vi "ifr2025 Sweep Mode.vi"(5 "Sweep Type (Linear)":bool=TRUE, 6 "Trigger Source (Front Panel)":i16(ring)=10 items=["Hold", "TTLTRG0", "TTLTRG1", "TTLTRG2", "TTLTRG3", "TTLTRG4", "TTLTRG5", "TTLTRG6", "TTLTRG7", "BUS", "Front Panel"], 7 "Trigger mode (Start Only)":i16(ring)=1 items=["Off", "Start Only", "Start / Stop", "Step"], 8 "error in (no error)":errorcluster {"code" format="%.0x"}, 9 "Sweep Mode (Single)":bool=TRUE, 10 "Carr Freq (Fixed)":bool=TRUE, 11 "instrument handle":refnum<visa-resource-name>) -> (0 "error out":errorcluster {"code" format="%.0x"}, 3 "instrument handle out":refnum<visa-resource-name>)   [LabVIEW 2009]
doc: "This command defines the carrier mode (SWEPT or FIXED) and the remainder of the SWEPT mode parameters."
uses:
  Ifr2025_32.dll
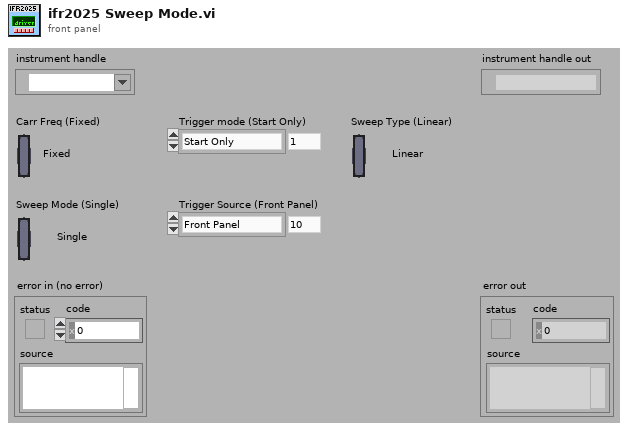
[diagram p1: front panel]
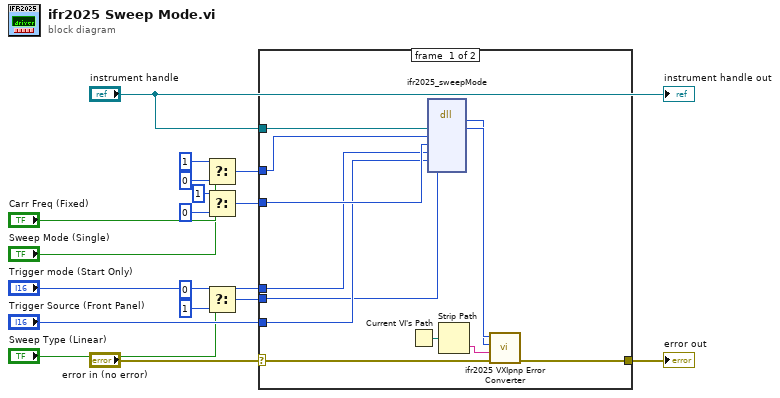
[diagram p0: block diagram]
diagram:
  n1 = Select(t=i16 1, s="Carr Freq (Fixed)", f=i16 0) -> (s? t:f=w11:i16)
  n2 = Select(t=i16 1, s="Sweep Mode (Single)", f=i16 0) -> (s? t:f=w7:i16)
  n3 = Select(t=i16 0, s="Sweep Type (Linear)", f=i16 1) -> (s? t:f=w1:i16)
  n4 = case shown="No Error" "error in (no error)" {
    selector: "error in (no error)" -> [w24 w30]
    tunnel: [w23 w30] -> w17
    tunnel: "instrument handle" -> [w28 _]
    tunnel: w11 -> [w22 _]
    tunnel: w7 -> [w21 _]
    tunnel: "Trigger mode (Start Only)" -> [w20 _]
    tunnel: "Trigger Source (Front Panel)" -> [w19 _]
    tunnel: w1 -> [w18 _]
    frame #0 {
      n5 = Current VI's Path() -> (path=w29:path)
      n6 = dll-call lib="P:/inst/Marconi 2024 Signal Generator/source/labview/ifr2025/ifr2025/ifr2025_*.*" fn="ifr2025_sweepMode"("vi"=w28, "Carr Freq"=w22, "Sweep Mode"=w21, "Trigger mode"=w20, "Trigger Source"=w19, "Sweep Type"=w18) -> (w26:i32, "vi"=w27:u32)  [unwired: 8 in, 2 out]
      n7 = Strip Path(path=w29) -> (name=w25:string)  [unwired: 1 out]
      n8 = call "ifr2025 VXIpnp Error Converter.vi"("error in (no error)"=w24, "name of VI (\"\")"=w25, "CVI error code (0)"=w26, "instrument handle"=w27) -> ("error out"=w23:errorcluster)  [unwired: 7 out]
    }
    frame #1 {
    }
  }
  "error out" <- w17
  "instrument handle out" <- "instrument handle"
